vi "数值输入窗口.vi"(0 "为真忽略上下限":bool, 1 "消息入队":refnum<queue>, 2 "字符串":string, 3 "字符消息入队列":string, 5 "输入下限":dbl, 7 "输入上限":dbl, 9 "转换比例":u32=1 min=1 max=1000000, 11 "数据类型":enum16{"32位", "16位"}(ring), 13 "控件引用":refnum<vi>) -> (4 "输出":bool, 6 "十六位":i16, 8 "32位":i32)   [LabVIEW 2018]
panel:
  in  "选项卡控件":enum32{"选项卡 1", "选项卡 2"}(tab)
  in  "输入框":dbl
  in  "确定按钮":bool
  in  "取消按钮":bool
  # "上限值"
  # "下限值"
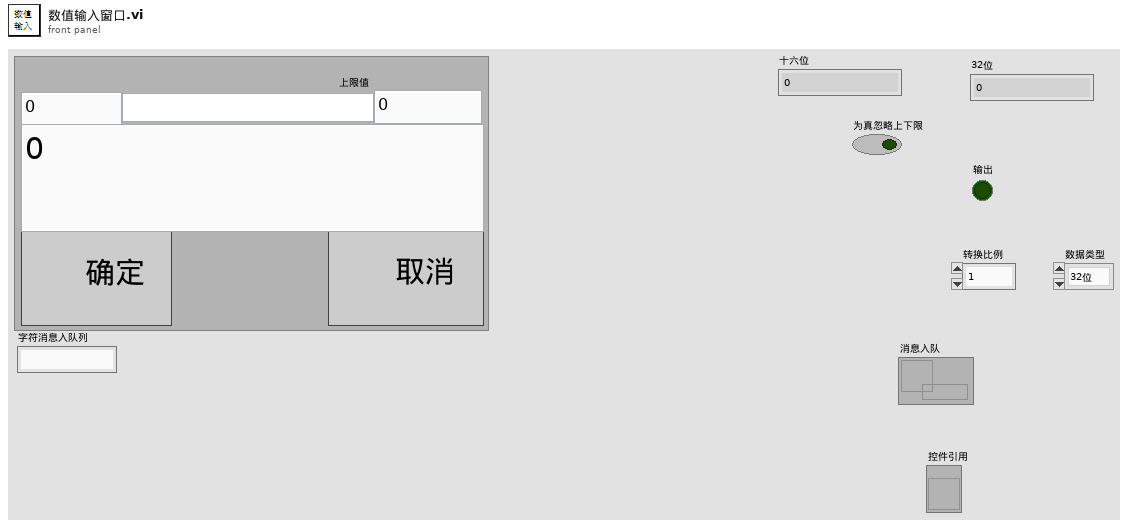
[diagram p1: front panel]
types:
  T1 = enum8{"Enabled", "Disabled", "Disabled and Grayed Out"}
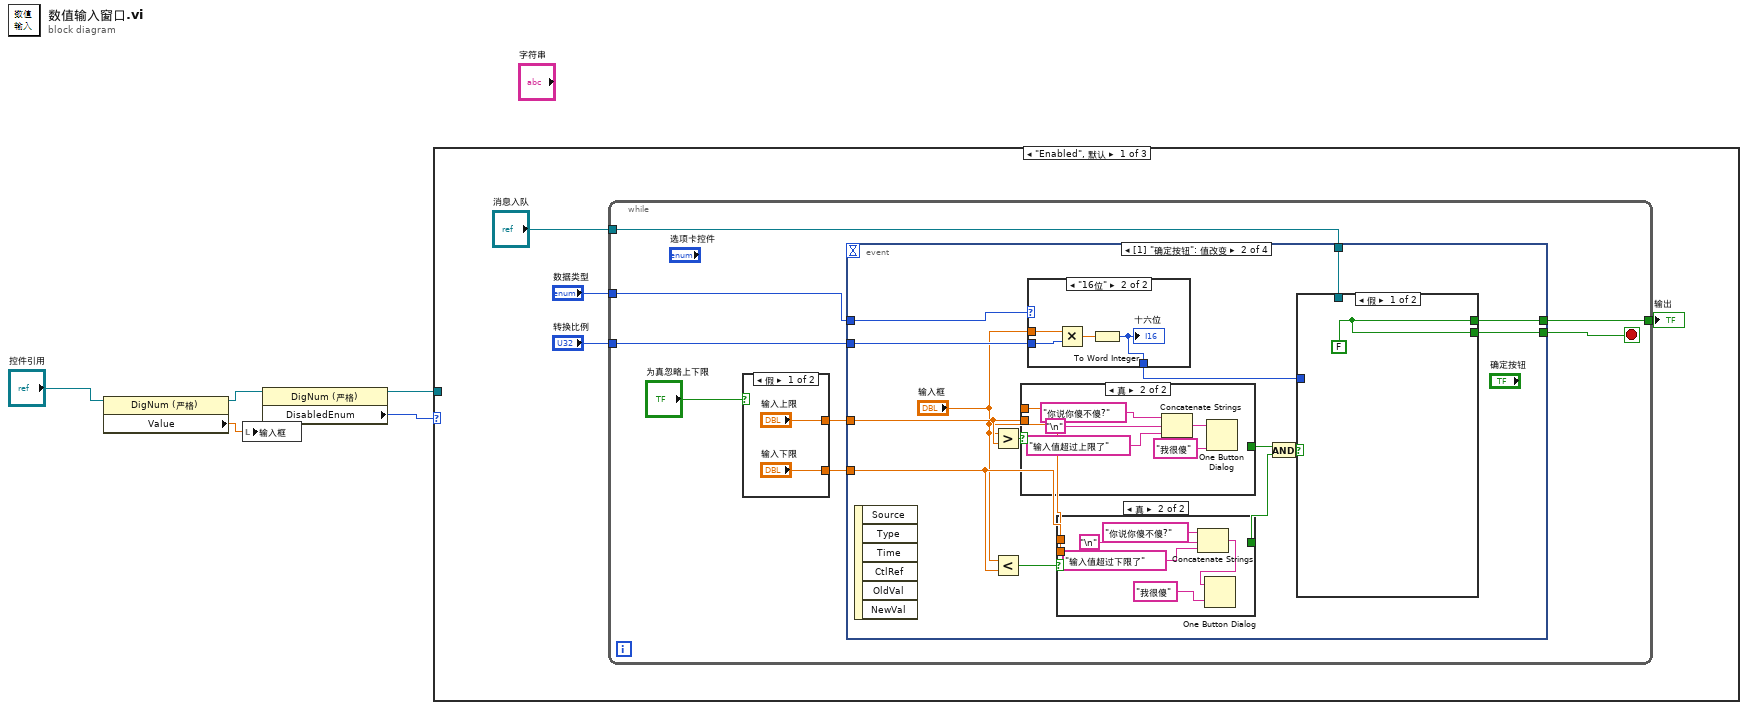
[diagram p0: block diagram]
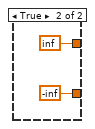
[diagram p2: hidden frame]
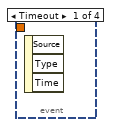
[diagram p3: hidden frame]
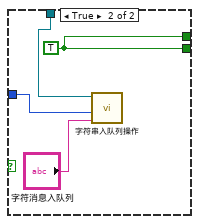
[diagram p4: hidden frame]
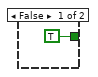
[diagram p5: hidden frame]
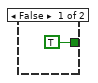
[diagram p6: hidden frame]
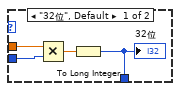
[diagram p7: hidden frame]
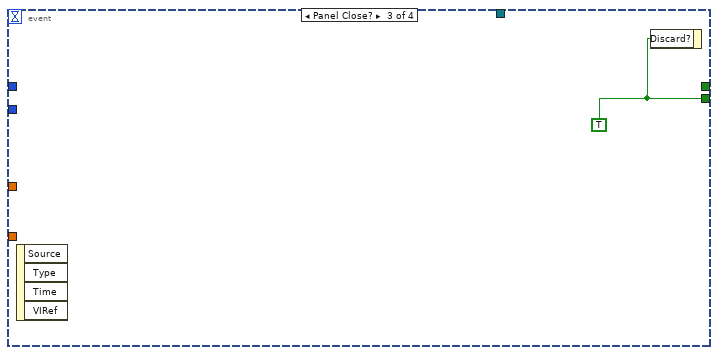
[diagram p8: hidden frame]
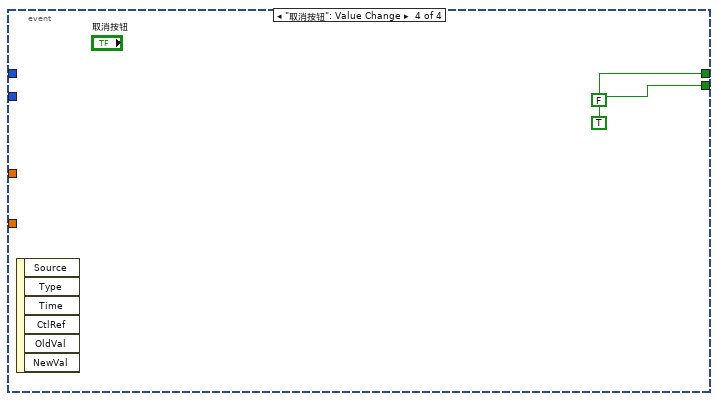
[diagram p9: hidden frame]
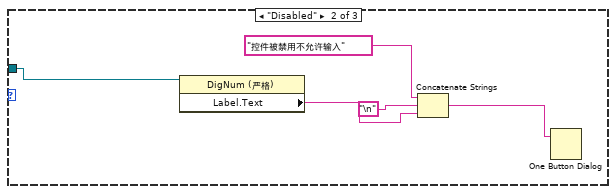
[diagram p10: hidden frame]
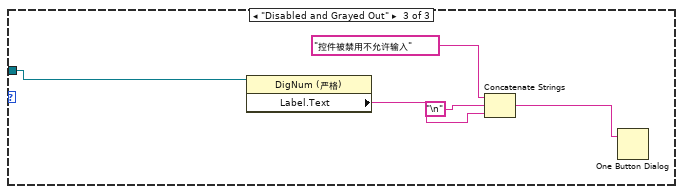
[diagram p11: hidden frame]
diagram:
  n1 = property class="DigNum (严格)"(reference="控件引用") -> (reference out=w2:refnum<vi>, "Value"=w4:dbl)  [unwired: 1 in, 1 out]
  n2 = local write "输入框"(w4) -> ()
  n3 = property class="DigNum (严格)"(reference=w2) -> (reference out=w1:refnum<vi>, "DisabledEnum"=w5:T1)  [unwired: 1 in, 1 out]
  n4 = case shown="\"Enabled\", 默认" w5 {
    tunnel: w1 -> [_ w66 w69]
    frame "Enabled", Default {
      n5 = while {
        tunnel: [w16] -> w9
        tunnel: "数据类型" -> [w15]
        tunnel: "转换比例" -> [w14]
        tunnel: "消息入队" -> [w10]
        stop <- w17 stop-if-true
        n6 = case shown="假" "为真忽略上下限" {
          tunnel: ["输入上限" inf] -> w12
          tunnel: ["输入下限" -inf] -> w11
          frame False {
          }
          frame True {
          }
        }
        n7 = event shown="[1] \"确定按钮\": 值改变" {
          selector: _ -> [_ _ _ _]
          dyn-events: _ -> [_ _ _ _]
          timeout: _ -> [_ _ _ _]
          tunnel: [_ w27 w61 TRUE] -> w17
          tunnel: [_ w25 _ FALSE] -> w16
          tunnel: w15 -> [_ w35 _ _]
          tunnel: w14 -> [_ w26 _ _]
          tunnel: w12 -> [_ w32 _ _]
          tunnel: w11 -> [_ w31 _ _]
          tunnel: w10 -> [_ w23 _ _]
          event Timeout {
            n8 = event-data() -> ()  [unwired: 1 in, 3 out]
          }
          event "确定按钮": Value Change {
            n9 = event-data() -> ()  [unwired: 1 in, 6 out]
            n10 = Greater?(x="输入框", y=w32) -> (0:w34:bool)
            n11 = Less?(x="输入框", y=w31) -> (x < y?=w33:bool)
            n12 = case shown="真" w34 {
              tunnel: "输入框" -> [_ _]
              tunnel: w32 -> [_ _]
              tunnel: [TRUE _] -> w30
              frame False {
              }
              frame True {
                n13 = Concatenate Strings("你说你傻不傻?" ("字符串"), "\n", "输入值超过上限了" ("消息")) -> (w51:string)
                n14 = One Button Dialog(message=w51, button name ("OK")="我很傻" ("按钮名称（“确定”）")) -> ()  [unwired: 1 out]
              }
            }
            n15 = case shown="\"16位\"" w35 {
              tunnel: w26 -> [w54 w60]
              tunnel: "输入框" -> [w55 w59]
              tunnel: [w53 w57] -> w22
              frame "32位", Default {
                n16 = Multiply(x=w55, y=w54) -> (x*y=w56:dbl)
                n17 = To Long Integer(number=w56) -> (32bit integer=w53:i32)
                "32位" <- w53
              }
              frame "16位" {
                n18 = Multiply(x=w59, y=w60) -> (x*y=w58:dbl)
                n19 = To Word Integer(number=w58) -> (16bit integer=w57:i16)
                "十六位" <- w57
              }
            }
            n20 = case shown="真" w33 {
              tunnel: "输入框" -> [_ _]
              tunnel: w31 -> [_ _]
              tunnel: [TRUE _] -> w29
              frame False {
              }
              frame True {
                n21 = Concatenate Strings("你说你傻不傻?" ("字符串"), "\n", "输入值超过下限了" ("消息")) -> (w42:string)
                n22 = One Button Dialog(message=w42, button name ("OK")="我很傻" ("按钮名称（“确定”）")) -> ()  [unwired: 1 out]
              }
            }
            n23 = And(x=w30, y=w29) -> (x .and. y?=w28:bool)
            n24 = case shown="假" w28 {
              tunnel: [w36 w40] -> w27
              tunnel: [w36 w40] -> w25
              tunnel: w23 -> [_ w39]
              tunnel: w22 -> [_ w38]
              frame False {
                w36 = FALSE
              }
              frame True {
                w40 = TRUE
                n25 = call "字符串入队列操作.vi"("字符消息入队列"="字符消息入队列", "数值"=w38, "界面切换队列"=w39) -> ()  [unwired: 8 in, 1 out]
              }
            }
          }
          event Panel Close? {
            w61 = TRUE ("放弃？")
            n26 = event-data() -> ()  [unwired: 1 in, 4 out]
            n27 = event-data("Discard?"=w61) -> ()  [unwired: 1 in, 1 out]
          }
          event "取消按钮": Value Change {
            n28 = event-data() -> ()  [unwired: 1 in, 6 out]
          }
        }
      }
      "输出" <- w9
    }
    frame "Disabled" {
      n29 = property class="DigNum (严格)"(reference=w66) -> ("Label.Text"=w64:string)  [unwired: 1 in, 2 out]
      n30 = Concatenate Strings("控件被禁用不允许输入" ("字符串"), "\n", w64) -> (w67:string)
      n31 = One Button Dialog(message=w67) -> ()  [unwired: 1 in, 1 out]
    }
    frame "Disabled and Grayed Out" {
      n32 = property class="DigNum (严格)"(reference=w69) -> ("Label.Text"=w70:string)  [unwired: 1 in, 2 out]
      n33 = Concatenate Strings("控件被禁用不允许输入" ("字符串"), "\n", w70) -> (w72:string)
      n34 = One Button Dialog(message=w72) -> ()  [unwired: 1 in, 1 out]
    }
  }
